vi "Data (Global).vi"(0 "Data In":dbl[](array[numeric]), 2 "Mode":T1(ring), 9 "Slope":dbl[](array[numeric]), 11 "Offset":dbl[](array[numeric]), 12 "Write Stream Error":errorcluster) -> (4 "Data Out":dbl[][](array[numeric]), 8 "New Data":bool, 10 "OverwriteErr#":i32, 15 "StreamErr#":i32)   [LabVIEW 2013]
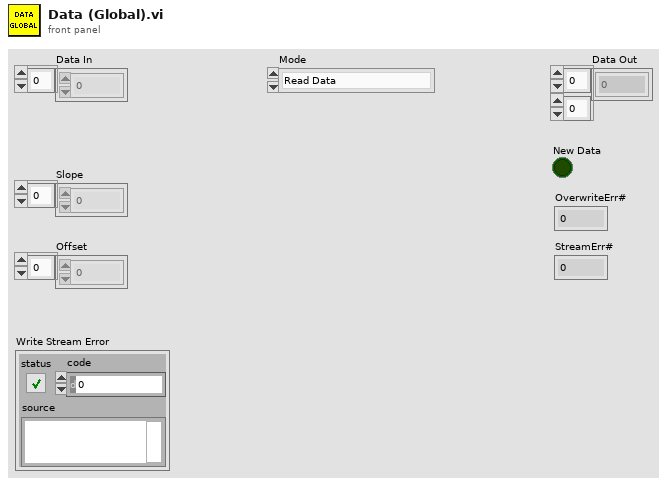
[diagram p1: front panel]
types:
  T1 = enum16{"Read Data", "Write Data", "Write Cal", "Init", "Write Stream Error"}
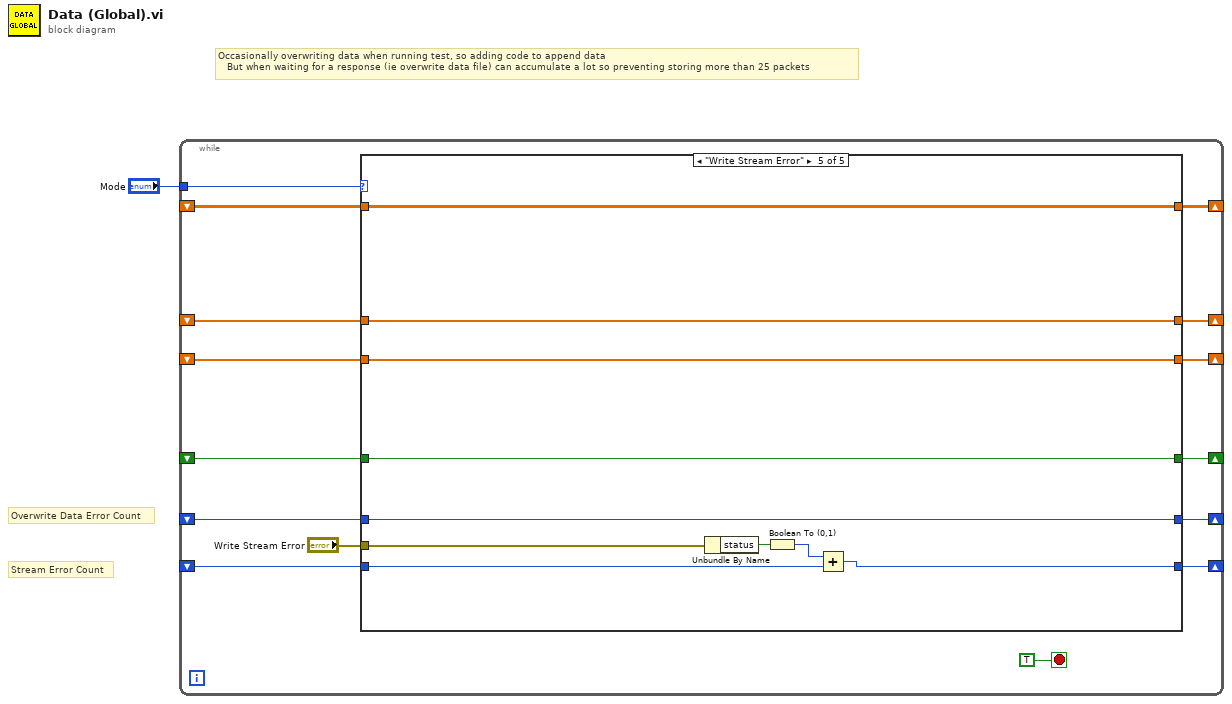
[diagram p0: block diagram]
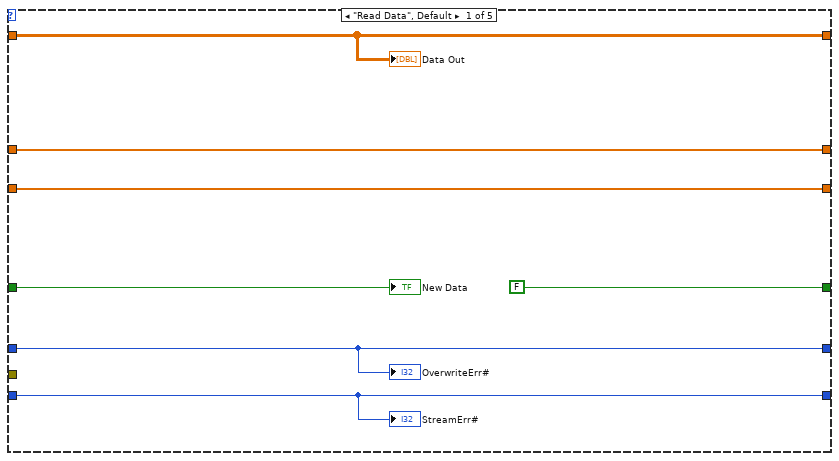
[diagram p2: hidden frame]
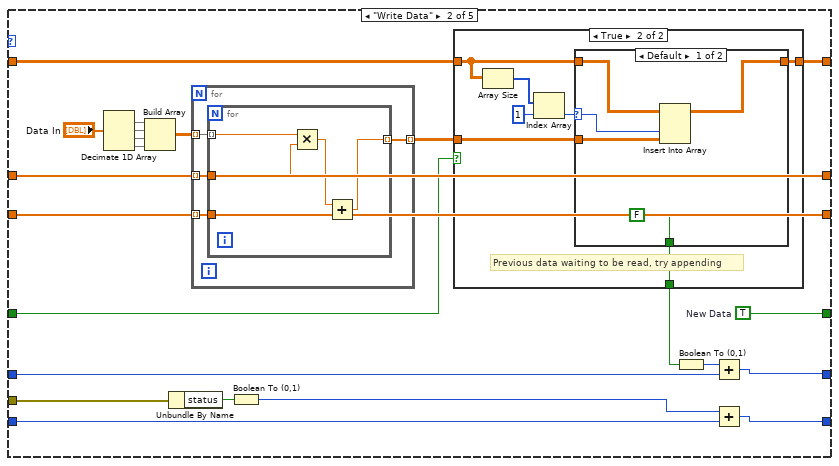
[diagram p3: hidden frame]
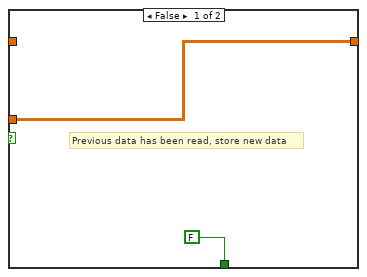
[diagram p4: hidden frame]
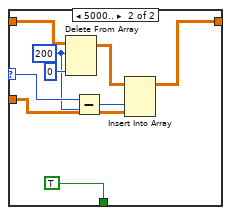
[diagram p5: hidden frame]
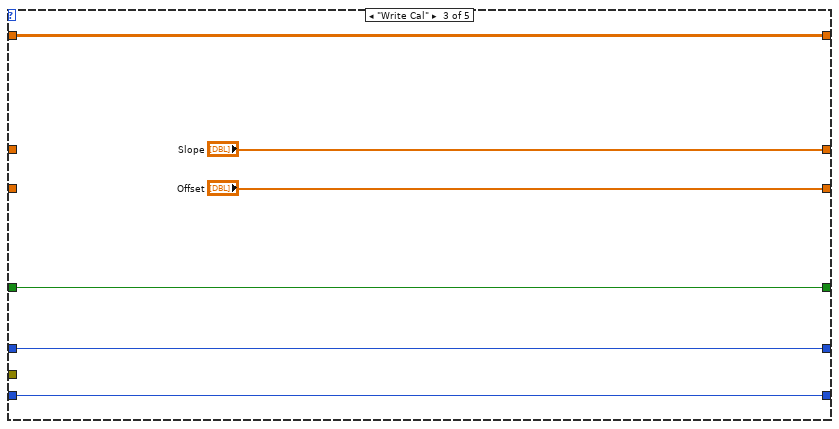
[diagram p6: hidden frame]
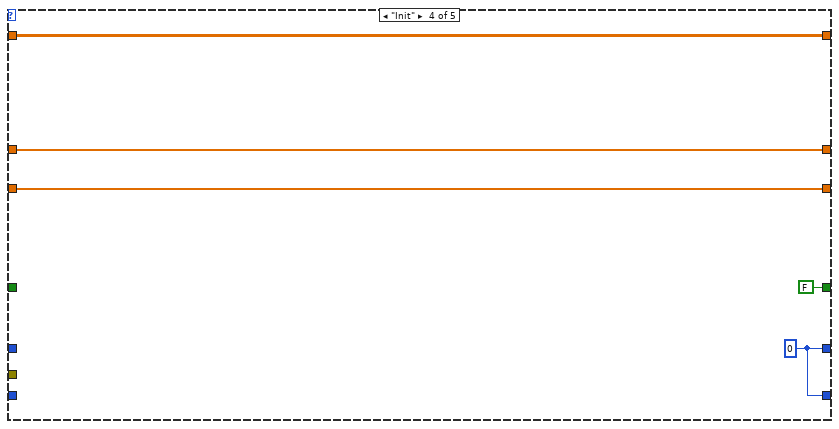
[diagram p7: hidden frame]
diagram:
  # "Stream Error Count"
  # "Overwrite Data Error Count"
  # "Occasionally overwriting data when running test, so adding code to append data\n   But when waiting for a response (ie overwrite data file) can accumulate a lot so preventing storing more than 25 packets"
  n1 = while {
    tunnel: "Mode" -> [w15]
    shift-right: [w14] -> _
    shift-left: _ -> [w13]
    shift-right: [w11] -> _
    shift-left: _ -> [w9]
    shift-right: [w12] -> _
    shift-left: _ -> [w10]
    shift-right: [w8] -> _
    shift-left: _ -> [w7]
    shift-right: [w6] -> _
    shift-left: _ -> [w4]
    shift-right: [w5] -> _
    shift-left: _ -> [w3]
    stop <- TRUE stop-if-true
    n2 = case shown="\"Write Stream Error\"" w15 {
      tunnel: [w21 w34 w81 w88 w98] -> w14
      tunnel: w13 -> [w21 w33 w81 w88 w98]
      tunnel: [w23 w38 "Slope" w87 w97] -> w12
      tunnel: [w22 w39 "Offset" w86 w96] -> w11
      tunnel: w10 -> [w23 w38 _ w87 w97]
      tunnel: w9 -> [w22 w39 _ w86 w96]
      tunnel: [FALSE ("New Data") w37 w80 FALSE ("New Data") w94] -> w8
      tunnel: w7 -> [w19 w36 w80 _ w94]
      tunnel: [w18 w30 w79 w84 w95] -> w6
      tunnel: [w17 w27 w78 w84 w90] -> w5
      tunnel: w4 -> [w18 w28 w79 _ w95]
      tunnel: w3 -> [w17 w25 w78 _ w89]
      tunnel: "Write Stream Error" -> [_ w24 _ _ w92]
      frame "Read Data", Default {
        "Data Out" <- w21
        "New Data" <- w19
        "OverwriteErr#" <- w18
        "StreamErr#" <- w17
      }
      frame "Write Data" {
        w37 = TRUE  # New Data
        n3 = Decimate 1D Array("Data In") -> (w42:dbl[], w43:dbl[], w44:dbl[], w45:dbl[])  [unwired: 1 out]
        n4 = Build Array(w42, w43, w44, w45) -> (w40:dbl[][])
        n5 = Unbundle By Name(w24) -> ("status"=w32:bool)
        n6 = for {
          tunnel: w40 -> [w70] mode=indexing
          tunnel: w38 -> [w72] mode=indexing
          tunnel: w39 -> [w71] mode=indexing
          tunnel: [w69] -> w35 mode=indexing
          n7 = for {
            tunnel: w72 -> [w76]
            tunnel: w71 -> [w75]
            tunnel: w70 -> [w77] mode=indexing
            tunnel: [w73] -> w69 mode=indexing
            n8 = Multiply(x=w77, y=w76) -> (x*y=w74:dbl)
            n9 = Add(x=w74, y=w75) -> (x+y=w73:dbl)
          }
        }
        n10 = Boolean To (0,1)(Boolean=w32) -> (0, 1=w26:i16)
        n11 = case shown="True" w36 {
          tunnel: w35 -> [w47 w50]
          tunnel: [w47 w49] -> w34
          tunnel: w33 -> [_ w51]
          tunnel: [FALSE w48] -> w31
          frame False {
            # "Previous data has been read, store new data"
          }
          frame True {
            # "Previous data waiting to be read, try appending"
            n12 = Array Size(array=w51) -> (size(s)=w54:i32[])
            n13 = Index Array(array=w54, index=1) -> (element=w52:i32)
            n14 = case shown="Default" w52 {
              selector: w52 -> [w58 w63]
              tunnel: w51 -> [w59 w68]
              tunnel: w50 -> [w57 w65]
              tunnel: [w56 w64] -> w49
              tunnel: [FALSE TRUE] -> w48
              frame Default {
                n15 = Insert Into Array(array=w59, index (col)=w58, new element=w57) -> (w56:dbl[][])  [unwired: 1 in]
              }
              frame 5000.. {
                w62 = 200 ("length")
                n16 = Delete From Array(array=w68, length=w62, index (col)=0 ("disabled index (col)")) -> (array with subset deleted=w66:dbl[][])  [unwired: 1 in, 1 out]
                n17 = Subtract(x=w63, y=w62) -> (x-y=w61:i32)
                n18 = Insert Into Array(array=w66, index (col)=w61, new element=w65) -> (w64:dbl[][])  [unwired: 1 in]
              }
            }
          }
        }
        n19 = Boolean To (0,1)(Boolean=w31) -> (0, 1=w29:i16)
        n20 = Add(x=w29, y=w28) -> (x+y=w30:i32)
        n21 = Add(x=w26, y=w25) -> (x+y=w27:i32)
      }
      frame "Write Cal" {
      }
      frame "Init" {
        w84 = 0
      }
      frame "Write Stream Error" {
        n22 = Unbundle By Name(w92) -> ("status"=w93:bool)
        n23 = Boolean To (0,1)(Boolean=w93) -> (0, 1=w91:i16)
        n24 = Add(x=w91, y=w89) -> (x+y=w90:i32)
      }
    }
  }
